vi "SwerveLatchGoalAngle.vi"(1 "Raw Goal Angle":dbl format="%#_13g", 2 "In Deadband":bool) -> (0 "Latched Goal Angle":dbl)   [LabVIEW 2019]
doc: "Latches the goal azimuth angle when the driver releases the stick. This prevents the modules from slewing to a new orientation and jerking the robot."
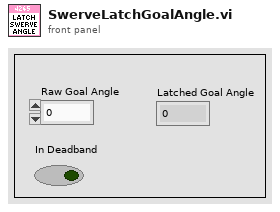
[diagram p1: front panel]
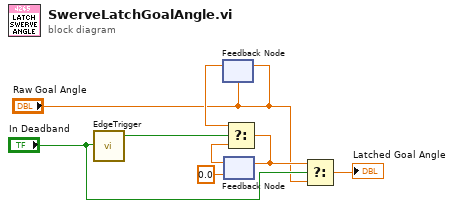
[diagram p0: block diagram]
diagram:
  n1 = call "EdgeTrigger.vi"("Input Signal"="In Deadband") -> ("Rising Edge Trigger"=w4:bool)  [unwired: 2 out]
  n2 = feedback-in #1("Raw Goal Angle") -> ()
  n3 = feedback #1("Raw Goal Angle") -> (w2:dbl)
  n4 = feedback #2(0.0 ("Raw Goal Angle")) -> (w5:dbl)
  n5 = Select(t=w2, s=w4, f=w5) -> (s? t:f=w6:dbl)
  n6 = feedback-in #2(w6) -> ()
  n7 = Select(t=w6, s="In Deadband", f="Raw Goal Angle") -> (s? t:f=→"Latched Goal Angle":dbl)
